vi "define_current_position_as_zero.vi"(8 "error in (no error)":errorcluster, 11 "Newport Model 8742 in":refnum<class "New Focus Model 8742.lvclass">) -> (0 "error out":errorcluster, 3 "Newport Model 8742 out":refnum<class "New Focus Model 8742.lvclass">)   [LabVIEW 2020, in "New Focus Model 8742.lvclass"]
uses:
  New Focus Model 8742.lvclass
  New Focus Model 8742.lvclass/New Focus Model 8742.ctl
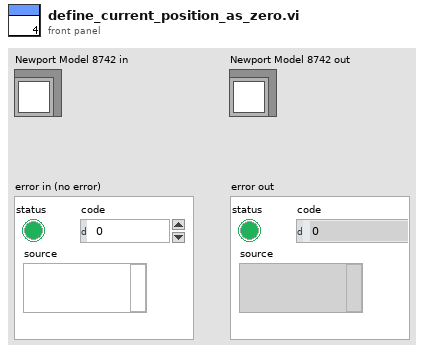
[diagram p1: front panel]
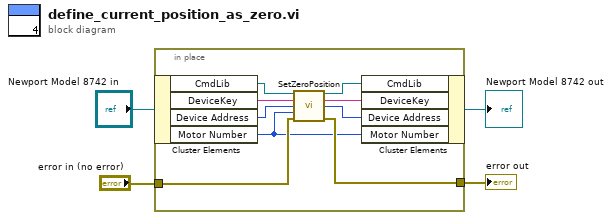
[diagram p0: block diagram]
diagram:
  n1 = in-place {
    in-place-border: "error in (no error)" -> [w10]
    in-place-border: [w9] -> w1
    n2 = in-place-cluster #1("Newport Model 8742 in") -> ("CmdLib"=w11:refnum<k24>, "DeviceKey"=w13:string, "Device Address"=w12:i32, "Motor Number"=w8:i32)
    n3 = call <instrlib>:"SetZeroPosition.vi"("CmdLib In"=w11, "DeviceKey In"=w13, "Device Address In"=w12, "Motor"=w8, "error in (no error)"=w10) -> ("CmdLib Out"=w5:refnum<k24>, "DeviceKey Out"=w6:string, "Device Address Out"=w7:i32, "error out"=w9:errorcluster)  [unwired: 7 in]
    n4 = in-place-cluster #1("CmdLib"=w5, "DeviceKey"=w6, "Device Address"=w7, "Motor Number"=w8) -> (→"Newport Model 8742 out":refnum<class "New Focus Model 8742.lvclass">)
  }
  "error out" <- w1
